vi "Set Process Variable Value - RSS.vi"(7 "Unit Address (1)":u8=1, 8 "error in (no error)":errorcluster, 9 "Process Variable  (0)":i32, 10 "Register Addresses (0)":i32=1, 11 "VISA resource name":refnum<visa-resource-name>) -> (0 "error out":errorcluster, 3 "VISA resource name out":refnum<visa-resource-name>)   [LabVIEW 2013, in "Eurotherm 35xx Series.lvlib"]
doc: "This VI sets Process Variable Value."
uses:
  <instrlib>/Eurotherm 35xx Series/Eurotherm 35xx Series.lvlib
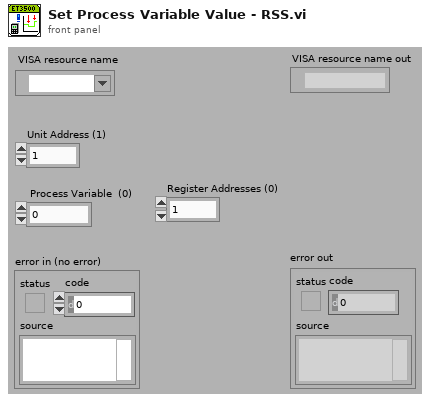
[diagram p1: front panel]
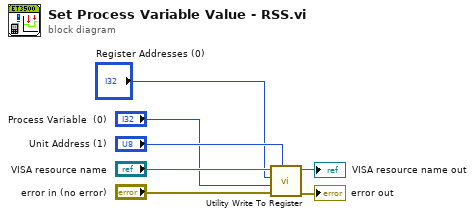
[diagram p0: block diagram]
diagram:
  n1 = call <instrlib>:"Utility Write To Register.vi"("Unit Address (1)"="Unit Address (1)", "error in (no error)"="error in (no error)", "Data (0)"="Process Variable  (0)", "Register Address (0)"="Register Addresses (0)", "VISA resource name"="VISA resource name") -> ("error out"=→"error out":errorcluster, "VISA resource name out"=→"VISA resource name out":refnum<visa-resource-name>)  [unwired: 5 in]
